vi "Write Port.vi"(0 "NXP in":refnum<class "NXP.lvclass">, 5 "VISA resource name":refnum<visa-resource-name>, 7 "Binary Number":T1, 9 "Port 2":dbl, 11 "error in (no error)":errorcluster) -> (4 "NXP out":refnum<class "NXP.lvclass">, 8 "VISA resource name 2":refnum<visa-resource-name>, 10 "Response":string, 15 "error out":errorcluster)   [LabVIEW 2020, in "NXP.lvclass"]
uses:
  NXP.lvclass
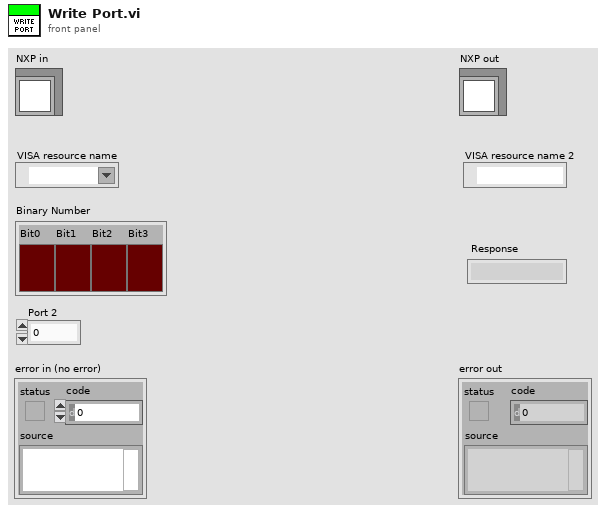
[diagram p1: front panel]
types:
  T1 = cluster{"Bit0":bool, "Bit1":bool, "Bit2":bool, "Bit3":bool}
  T2 = enum16{"Write", "Read", "Config", "Reset", "Close"}
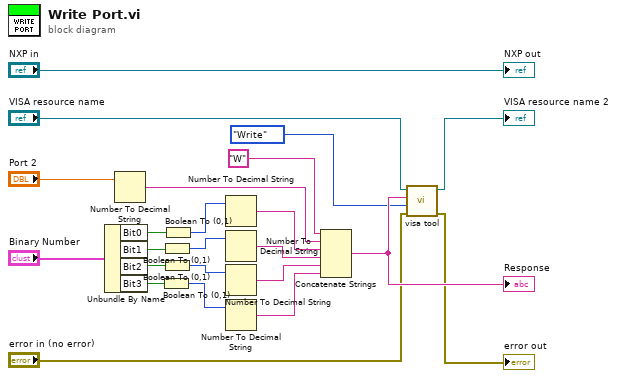
[diagram p0: block diagram]
diagram:
  n1 = Unbundle By Name("Binary Number") -> ("Bit0"=w22:bool, "Bit1"=w21:bool, "Bit2"=w20:bool, "Bit3"=w19:bool)
  n2 = Number To Decimal String(number="Port 2") -> (decimal integer string=w7:string)  [unwired: 1 in]
  n3 = Boolean To (0,1)(Boolean=w19) -> (0, 1=w17:i16)
  n4 = Boolean To (0,1)(Boolean=w21) -> (0, 1=w15:i16)
  n5 = Boolean To (0,1)(Boolean=w20) -> (0, 1=w16:i16)
  n6 = Boolean To (0,1)(Boolean=w22) -> (0, 1=w18:i16)
  n7 = Number To Decimal String(number=w18) -> (decimal integer string=w14:string)  [unwired: 1 in]
  n8 = Number To Decimal String(number=w15) -> (decimal integer string=w13:string)  [unwired: 1 in]
  n9 = Number To Decimal String(number=w16) -> (decimal integer string=w12:string)  [unwired: 1 in]
  n10 = Number To Decimal String(number=w17) -> (decimal integer string=w11:string)  [unwired: 1 in]
  n11 = Concatenate Strings("W" ("string"), w7, w14, w13, w12, w11) -> (w6:string)
  "Response" <- w6
  n12 = call "visa tool.vi"("error in (no error)"="error in (no error)", "Opciones"=T2."Write", "Write"=w6, "VISA com port"="VISA resource name") -> ("error out"=→"error out":errorcluster, "VISA com port 2"=→"VISA resource name 2":refnum<visa-resource-name>)  [unwired: 5 in, 1 out]
  "NXP out" <- "NXP in"
